vi "SplineHelp_GetQuinticCtrlVectorsFromWeightedWayPts_2762.vi"(9 "Use Weights":bool, 11 "WayPoints":T1[](array[typedef]) {"SCALAR" format="%14.3f"; "ROTATION"."SIN" format="%13.4f"; "ROTATION"."COS" format="%13.4f"; "ROTATION"."VALUE" format="%13.4f"; "TRANSLATION"."Y" format="%14.3f"; "TRANSLATION"."X" format="%14.3f"}) -> (3 "SplineControlVectors":T4[](array[typedef]))   [LabVIEW 2019]
doc: "Returns control vectors from a set of weighted waypoints. (I think this should be able to be used by Cubic splines too...)\n\nParameters:\n - Weighted Waypoints - The array of waypoints (Weighted WayPoint)\n - Use Weights -- Use the weight values if TRUE. Otherwise weights are ignored.\n\nReturns:\n - SplineControlVectors - Array of control vectors"
uses:
  SPLINE_CTRL_VECTOR.ctl
  WEIGHTED_WAYPOINT.ctl
  TRANSLATION2D.ctl
  ROTATION2D.ctl
  Trajectory_Library.lvlib
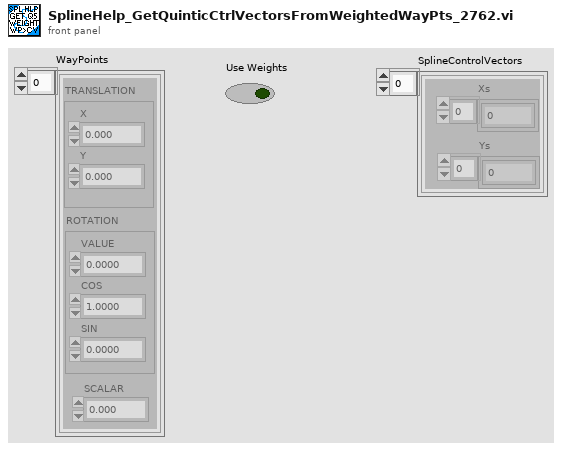
[diagram p1: front panel]
types:
  T1 = typedef "Trajectory_Library.lvlib/WEIGHTED_WAYPOINT.ctl" = cluster{"TRANSLATION":T2, "ROTATION":T3, "SCALAR":dbl}
  T2 = typedef "Trajectory_Library.lvlib/TRANSLATION2D.ctl" = cluster{"X":dbl, "Y":dbl}
  T3 = typedef "Trajectory_Library.lvlib/ROTATION2D.ctl" = cluster{"VALUE":dbl, "COS":dbl, "SIN":dbl}
  T4 = typedef "Trajectory_Library.lvlib/SPLINE_CTRL_VECTOR.ctl" = cluster{"Xs":dbl[], "Ys":dbl[]}
  T5 = typedef "Trajectory_Library.lvlib/POSE2D.ctl" = cluster{"TRANSLATION":T2, "ROTATION":T3}
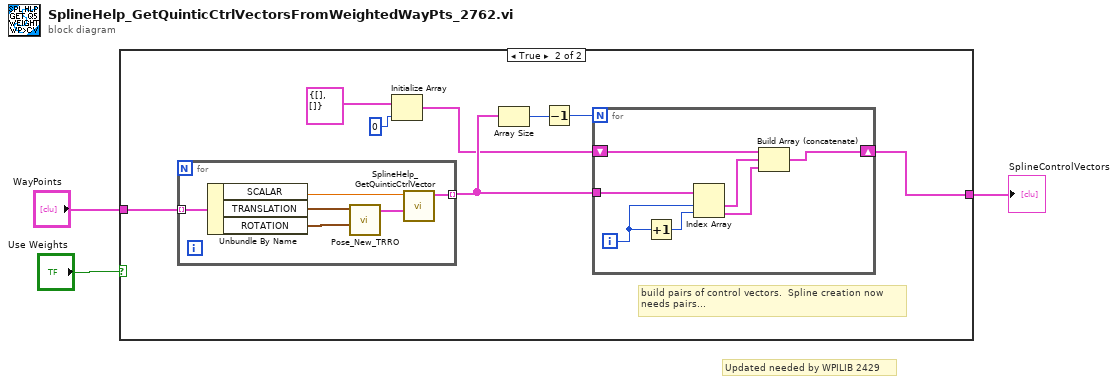
[diagram p0: block diagram]
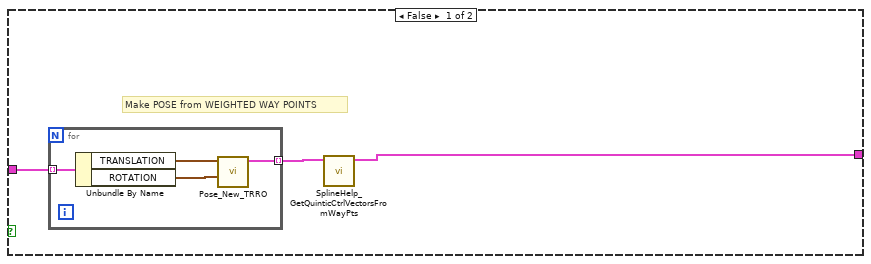
[diagram p2: hidden frame]
diagram:
  # "Updated needed by WPILIB 2429"
  n1 = case shown="True" "Use Weights" {
    tunnel: [w6 w11] -> w2
    tunnel: "WayPoints" -> [w5 w18]
    frame False {
      # "Make POSE from WEIGHTED WAY POINTS"
      n2 = for {
        tunnel: w5 -> [w10] mode=indexing
        tunnel: [w7] -> w4 mode=indexing
        n3 = Unbundle By Name(w10) -> ("TRANSLATION"=w9:T2, "ROTATION"=w8:T3)
        n4 = call "Pose_New_TRRO.vi"("ROTATION"=w8, "TRANSLATION"=w9) -> ("outPOSE"=w7:T5)  [unwired: 9 in]
      }
      n5 = call "SplineHelp_GetQuinticCtrlVectorsFromWayPts.vi"("WayPoints"=w4) -> ("SplineControlVectors"=w6:T4[])  [unwired: 10 in]
    }
    frame True {
      # "build pairs of control vectors.  Spline creation now\nneeds pairs..."
      n6 = for {
        tunnel: w18 -> [w31] mode=indexing
        tunnel: [w26] -> w15 mode=indexing
        n7 = Unbundle By Name(w31) -> ("SCALAR"=w27:dbl, "TRANSLATION"=w30:T2, "ROTATION"=w29:T3)
        n8 = call "Pose_New_TRRO.vi"("ROTATION"=w29, "TRANSLATION"=w30) -> ("outPOSE"=w28:T5)  [unwired: 9 in]
        n9 = call "SplineHelp_GetQuinticCtrlVector.vi"("Input POSE"=w28, "Scalar"=w27) -> ("resultSpline_Ctrl_Vector"=w26:T4)  [unwired: 9 in]
      }
      n10 = Initialize Array(T4 {"Xs"=[], "Ys"=[]} ("SPLINE_CTRL_VECTOR"), 0 ("dimension size")) -> (w12:T4[])
      n11 = Array Size(array=w15) -> (size(s)=w17:i32)
      n12 = Decrement(x=w17) -> (x-1=w16:i32)
      n13 = for {
        N: w16 -> [_]
        tunnel: w15 -> [w24]
        shift-right: [w19] -> w11
        shift-left: w12 -> [w22]
        i -> [w23]
        n14 = Increment(x=w23) -> (x+1=w25:i32)
        n15 = Index Array(array=w24, index #1=w23, index #2=w25) -> (element #1=w21:T4, element #2=w20:T4)
        n16 = Build Array (concatenate)(w22, w21, w20) -> (w19:T4[])
      }
    }
  }
  "SplineControlVectors" <- w2
